vi "LV_MD5.vi"(9 "error in (no error)":errorcluster, 10 "Input string":string) -> (1 "error out":errorcluster, 2 "MD5 digest (16-bytes)":string)   [LabVIEW 2023]
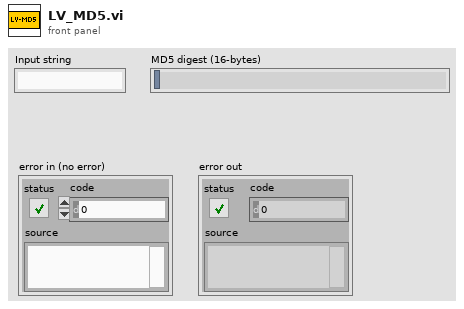
[diagram p1: front panel]
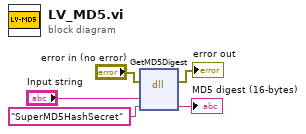
[diagram p0: block diagram]
diagram:
  n1 = dll-call lib="LabVIEW" fn="GetMD5Digest"(error in="error in (no error)", "InputString"="Input string", "MD5digest"="SuperMD5HashSecret") -> (error out=→"error out":errorcluster, "MD5digest"=→"MD5 digest (16-bytes)":string)  [unwired: 4 in, 1 out]
